vi "Write Names.vi"(8 "Value2 Name":string, 9 "Value1 Name":string, 10 "Effect Name":string, 11 "Effect Interface in":refnum<class "Effect Interface.lvclass">) -> (3 "Effect Interface out":refnum<class "Effect Interface.lvclass">)   [LabVIEW 2019, in "Effect Interface.lvlib" / "Effect Interface.lvclass"]
uses:
  Effect Interface.lvclass
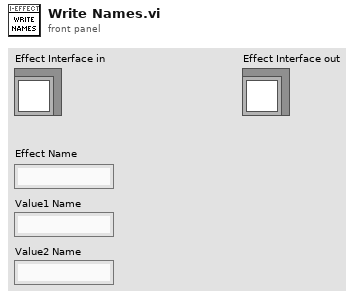
[diagram p1: front panel]
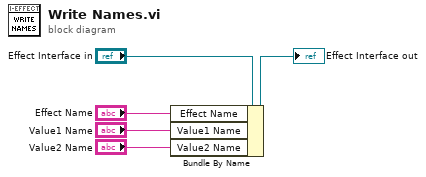
[diagram p0: block diagram]
diagram:
  n1 = Bundle By Name(cluster="Effect Interface in", "Effect Name"="Effect Name", "Value1 Name"="Value1 Name", "Value2 Name"="Value2 Name") -> (→"Effect Interface out":refnum<class "Effect Interface.lvclass">)
